vi "Test Suite.Serialize - Invalid character in Name - XML does not contain invalid character.vi"() -> ()   [LabVIEW 2013, in "JUnit XML Tests.lvlib"]
uses:
  JUnit XML Tests.lvlib
  <vilib>/xml/Close Reference(Node).vi
  <vilib>/addons/_JKI Toolkits/Caraya/classes/Assert/Assert Equal Value_Variant.vi
  JUnit XML/JUnit XML.lvlib
  JUnit XML/Test Suite/Test Suite.lvclass
  <vilib>/addons/_JKI Toolkits/Caraya/classes/Test/Test.lvclass
  <vilib>/addons/_JKI Toolkits/Caraya/classes/Assert/Assert.lvclass
  <resource>/objmgr/DOMUserDefRef.rc
  <vilib>/xml/NI_XML.lvlib
panel:
  out "error out":errorcluster
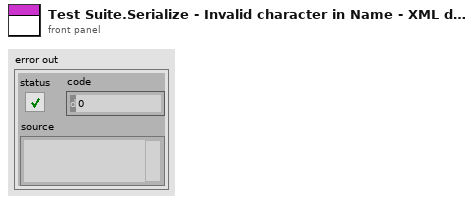
[diagram p1: front panel]
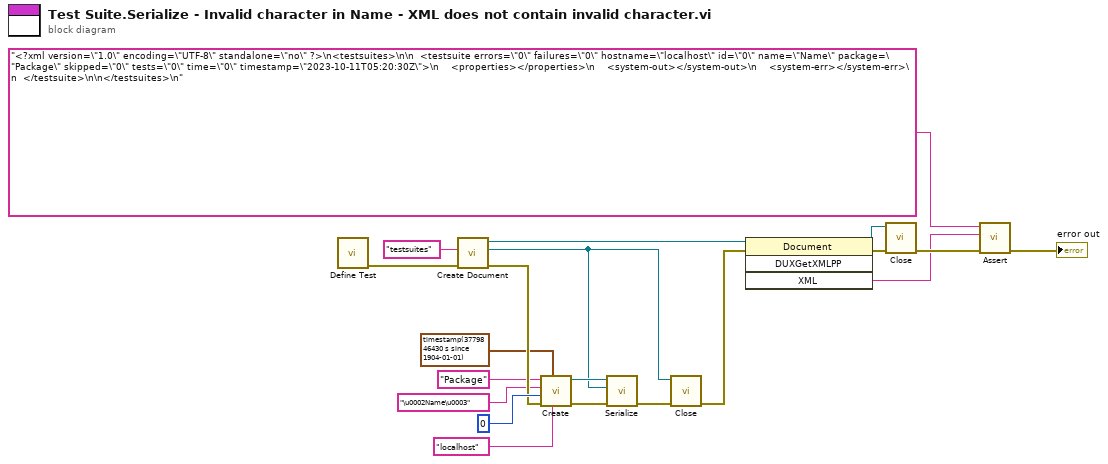
[diagram p0: block diagram]
diagram:
  n1 = call <vilib>:"Define Test.vi"() -> ("error out"=w20:errorcluster)  [unwired: 10 in, 1 out]
  n2 = call "Create Document.vi"("error in (no error)"=w20, "Root Element Name"="testsuites") -> ("error out"=w15:errorcluster, "Root Element"=w11:refnum<k20>, "Document"=w14:refnum<k20>)  [unwired: 7 in]
  n3 = call "Create.vi"("Hostname (\"localhost\")"="localhost" ("Package"), "Timestamp"=timestamp(3779846430.123 s since 1904-01-01), "error in (no error)"=w15, "Id"=0, "Name"="\u0002Name\u0003" ("Package"), "Package"="Package") -> ("error out"=w18:errorcluster, "Test Suite"=w19:refnum<class "Test Suite.lvclass">)  [unwired: 4 in]
  n4 = call "Serialize.vi"("error in (no error)"=w18, "Element in"=w11, "Test Suite in"=w19) -> ("error out"=w13:errorcluster)  [unwired: 7 in, 1 out]
  n5 = call-poly <vilib>:"Close.vi"("error in (no error)"=w13, "node"=w11) -> ("error out"=w12:errorcluster)  [unwired: 7 in]
  n6 = invoke class="Document" method="DUXGetXMLPP"(reference=w14, error in=w12) -> (reference out=w9:refnum<k20>, error out=w10:errorcluster, "XML"=w7:string)  [unwired: 2 in, 1 out]
  n7 = call-poly <vilib>:"Close.vi"("error in (no error)"=w10, "node"=w9) -> ("error out"=w8:errorcluster)  [unwired: 7 in]
  n8 = call-poly <vilib>:"Assert.vi"("error in (no error)"=w8, "Y"=w7, "X"="<?xml version=\"1.0\" encoding=\"UTF-8\" standalone=\"no\" ?>\n<testsuites>\n\n  <testsuite errors=\"0\" failures=\"0\" hostname=\"localhost\" id=\"0\" name=\"Name\" package=\"Package\" skipped=\"0\" tests=\"0\" time=\"0\" timestamp=\"2023-10-11T05:20:30Z\">\n    <properties></properties>\n    <system-out></system-out>\n    <system-err></system-err>\n  </testsuite>\n\n</testsuites>\n") -> ("error out"=→"error out":errorcluster)  [unwired: 7 in, 1 out]
